vi "myRIOXB Global.vi"() -> ()   [LabVIEW 2021]
doc: "This global variant stores information of Icon/Express VI name/Help/Error message for all myRIO Express VIs."
panel:
  in  "Context Help Separator":string="\r\n--------------------"
  in  "Invalid Channel Error Details":string="The current personality or target does not support the channels. Switch to another personality, change the current target, or open the Express VI to select supported channels."
  in  "Invalid Channel Error":string="The current personality or target does not support the channels."
  in  "Convert to subVI Button Name  (T)":string="Convert"
  in  "Convert to subVI Warn Message":string="Do you want to convert this Express VI to a standard subVI? You cannot view the configuration dialog box for this Express VI again."
  out "DO Block EVI Help Info":T1={"Description"="Writes values to one or more digital output channels. Use this Express VI to write multiple samples for each channel at one time.", "Path"=path "<helpdir>/myrioreference.chm", "Tag"="myrioref_exp_do.html"}
  in  "DO Block EVI Name":string="Digital output (n samples)"
  out "DO Block EVI Image":picture
  out "DI Block EVI Help Info":T1={"Description"="Reads values from one or more digital input channels. Use this Express VI to read multiple samples for each channel at one time.", "Path"=path "<helpdir>/myrioreference.chm", "Tag"="myrioref_exp_di.html"}
  out "DI Block EVI Image":picture
  in  "DI Block EVI Name":string="Digital input (n samples)"
  out "AO Block EVI Help Info":T1={"Description"="Writes values to one or more analog output channels. Use this Express VI to write multiple samples for each channel at one time.", "Path"=path "<helpdir>/myrioreference.chm", "Tag"="myrioref_exp_ao.html"}
  out "AO Block EVI Image":picture
  in  "AO Block EVI Name":string="Analog output (n samples)"
  out "AI Block EVI Help Info":T1={"Description"="Reads values from one or more analog input channels. Use this Express VI to read multiple samples for each channel at one time.", "Path"=path "<helpdir>/myrioreference.chm", "Tag"="myrioref_exp_ai.html"}
  out "AI Block EVI Image":picture
  in  "AI Block EVI Name":string="Analog input (n samples)"
  out "Audio Block Out EVI Help Info":T1={"Description"="Writes values to one or more audio output channels. Use this Express VI to write multiple samples for each channel at one time.", "Path"=path "<helpdir>/myrioreference.chm", "Tag"="myrioref_exp_audio_output_ns.html"}
  out "Encoder EVI Help Info":T1={"Description"="Reads and decodes signals from an encoder through the encoder channels. This Express VI reads the number of ticks that the encoder receives since the last counter reset.", "Path"=path "<helpdir>/myrioreference.chm", "Tag"="myrioref_exp_encoder.html"}
  out "DO EVI Help Info":T1={"Description"="Writes values to one or more digital output channels.", "Path"=path "<helpdir>/myrioreference.chm", "Tag"="myrioref_exp_do.html"}
  out "DI EVI Help Info":T1={"Description"="Reads values from one or more digital input channels.", "Path"=path "<helpdir>/myrioreference.chm", "Tag"="myrioref_exp_di.html"}
  out "Audio Block In EVI Help Info":T1={"Description"="Reads values from one or more audio input channels. Use this Express VI to read multiple samples for each channel at one time.", "Path"=path "<helpdir>/myrioreference.chm", "Tag"="myrioref_exp_audio_input_ns.html"}
  out "AO EVI Help Info":T1={"Description"="Writes values to one or more analog output channels.", "Path"=path "<helpdir>/myrioreference.chm", "Tag"="myrioref_exp_ao.html"}
  out "AI EVI Help Info":T1={"Description"="Reads values from one or more analog input channels.", "Path"=path "<helpdir>/myrioreference.chm", "Tag"="myrioref_exp_ai.html"}
  out "LED Help Info":T1={"Description"="Sets the states of the LEDs.", "Path"=path "<helpdir>/myrioreference.chm", "Tag"="myrioref_led.html"}
  out "Button EVI Help Info":T1={"Description"="Reads the value from the user programmable button.", "Path"=path "<helpdir>/myrioreference.chm", "Tag"="myrioref_button.html"}
  out "Accelerometer EVI Help Info":T1={"Description"="Reads acceleration values along the X, Y, and Z axes of the accelerometer.", "Path"=path "<helpdir>/myrioreference.chm", "Tag"="myrioref_accelerometer.html"}
  out "I2C EVI Help Info":T1={"Description"="Writes data to or reads data from an Inter-Integrated Circuit (I2C) slave device through the I2C channels.", "Path"=path "<helpdir>/myrioreference.chm", "Tag"="myrioref_exp_i2c.html"}
  out "PWM EVI Help Info":T1={"Description"="Generates a pulse width modulation (PWM) signal to an external peripheral through the PWM channels.", "Path"=path "<helpdir>/myrioreference.chm", "Tag"="myrioref_exp_pwm.html"}
  out "UART EVI Help Info":T1={"Description"="Writes data to or reads data from a Universal Asynchronous Receiver/Transmitter (UART) device through the UART channels. ", "Path"=path "<helpdir>/myrioreference.chm", "Tag"="myrioref_exp_uart.html"}
  out "SPI EVI Help Info":T1={"Description"="Writes data to or reads data from a serial peripheral interface (SPI) slave device through the SPI channels.", "Path"=path "<helpdir>/myrioreference.chm", "Tag"="myrioref_exp_spi.html"}
  out "IRQ EVI Help Info":T1={"Description"="Registers analog and digital input interrupts and creates timer interrupts.", "Path"=path "<helpdir>/myrioreference.chm", "Tag"="myrioref_exp_irq.html"}
  in  "IRQ EVI Name":string="Analog input interrupt"
  in  "LED EVI Name":string="LED"
  in  "Button EVI Name":string="Button"
  in  "UART EVI Name":string="UART"
  in  "DO EVI Name":string="Digital output (1 sample)"
  out "DO EVI Image":picture
  out "AI EVI Image":picture
  out "LED EVI Image":picture
  out "AO EVI Image":picture
  out "Audio Block In EVI Image":picture
  out "Audio Block Out EVI Image":picture
  out "DI EVI Image":picture
  out "Encoder EVI Image":picture
  out "I2C EVI Image":picture
  out "PWM EVI Image":picture
  out "SPI EVI Image":picture
  out "UART EVI Image":picture
  out "Button EVI Image":picture
  out "Accelerometer EVI Image":picture
  out "IRQ EVI Image":picture
  in  "Audio Block In EVI Name":string="Audio input (n samples)"
  in  "Audio Block Out EVI Name":string="Audio output (n samples)"
  in  "SPI EVI Name":string="SPI"
  in  "PWM EVI Name":string="PWM"
  in  "I2C EVI Name":string="I2C"
  in  "Encoder EVI Name":string="Encoder"
  in  "AO EVI Name":string="Analog output (1 sample)"
  in  "DI EVI Name":string="Digital input (1 sample)"
  in  "Accelerometer EVI Name":string="Accelerometer"
  in  "AI EVI Name":string="Analog input (1 sample)"
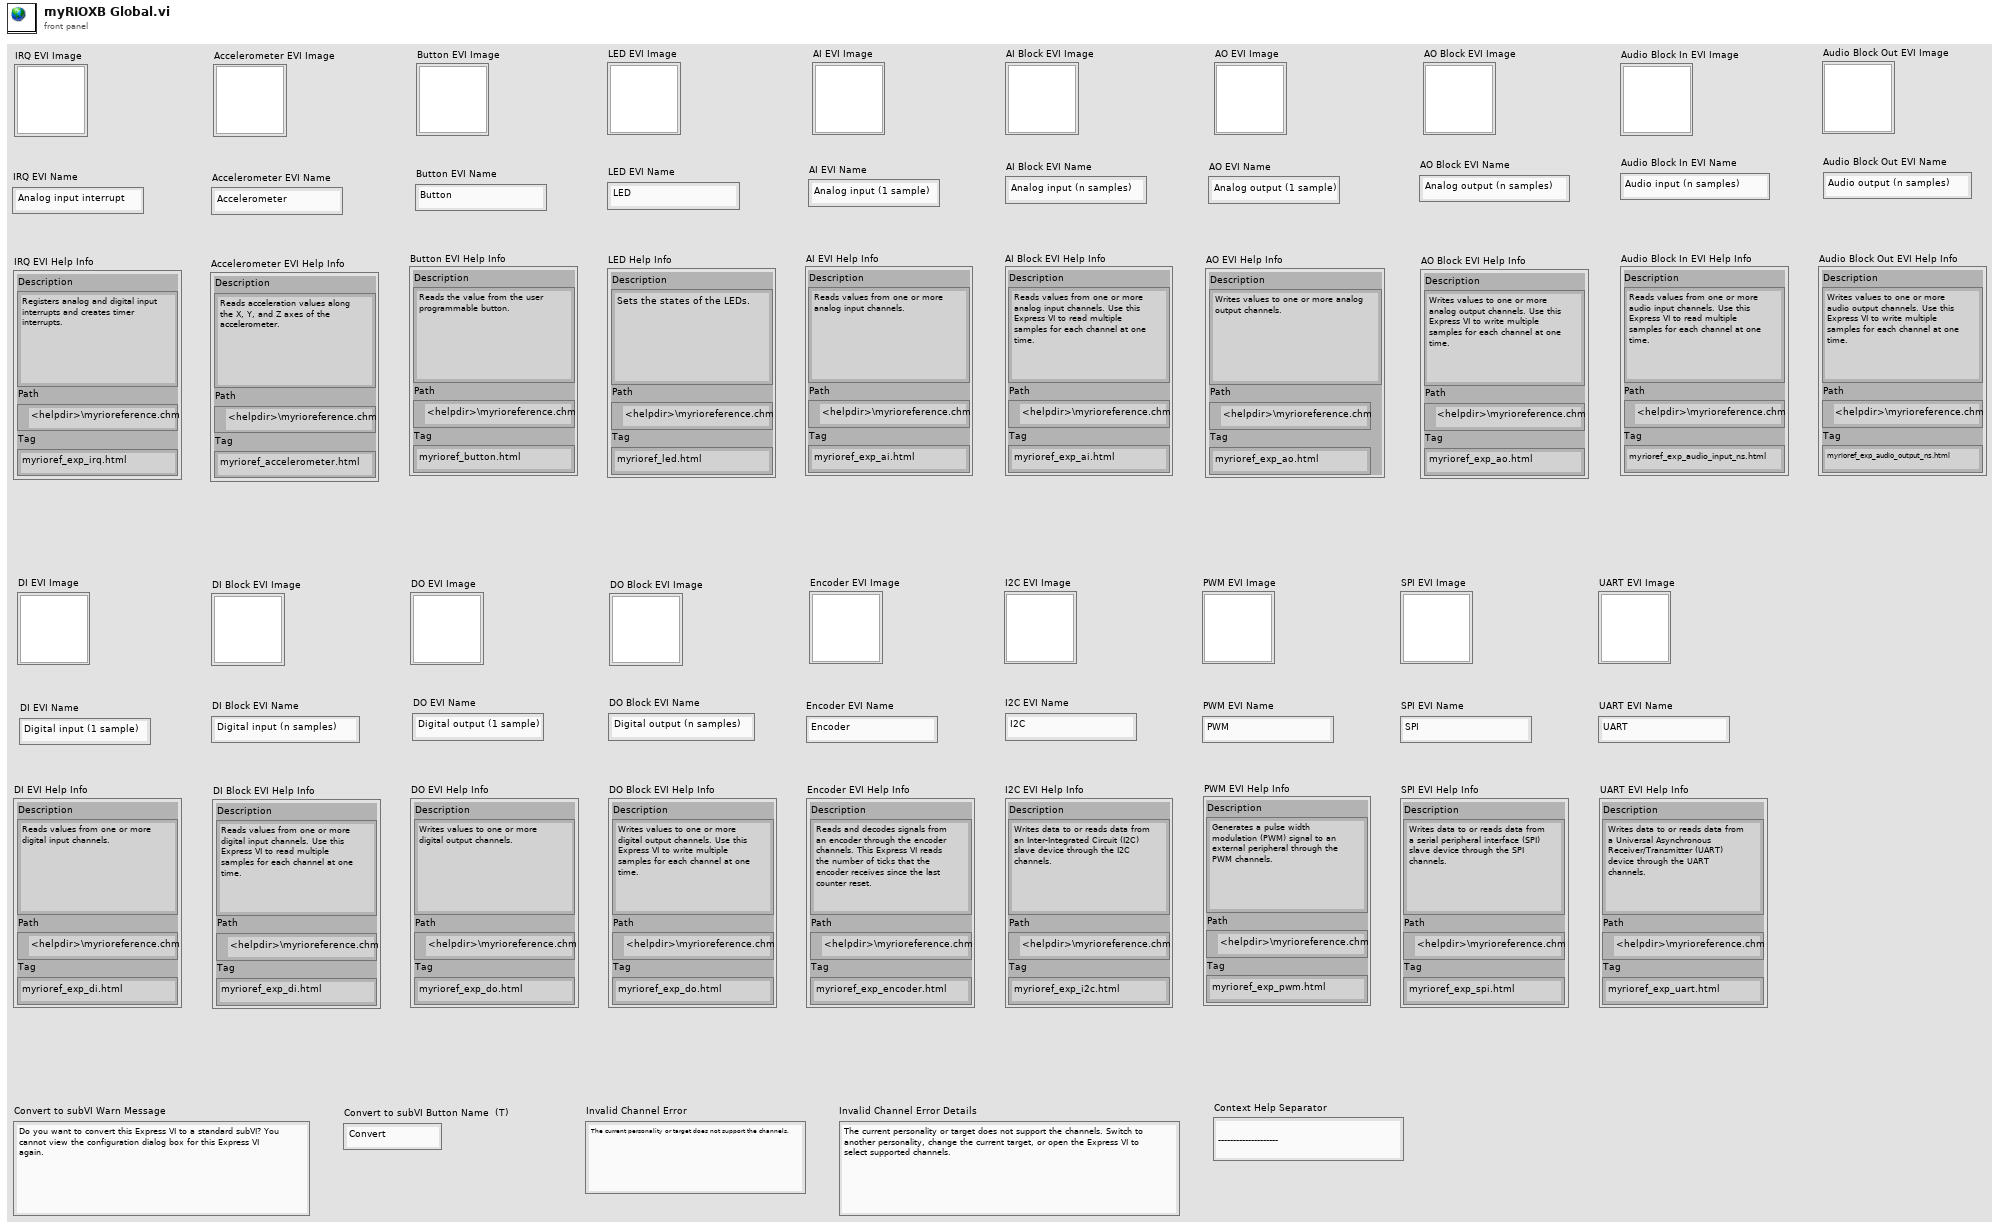
[diagram p1: front panel]
types:
  T1 = cluster{"Description":string, "Path":path, "Tag":string}
diagram:
